vi "BB_Remote Sense Test_v3.vi"(7 "error in (no error)":errorcluster, 10 "ControlBoard VISA":refnum<visa-resource-name>="ControlBoard") -> (0 "error out":errorcluster, 2 "Voltage Readings":dbl[][](array[numeric]), 3 "Pass?":bool)   [LabVIEW 2022 SP3]
panel:
  in  "RemoteSenseRelayTask":refnum<k21>="BTS_RemoteSenseRelays"
  out "Message OUT":string
  out "MSE Array":dbl[](array[numeric])
  in  "Message IN":string
  out "Control Board OUT":refnum<visa-resource-name>
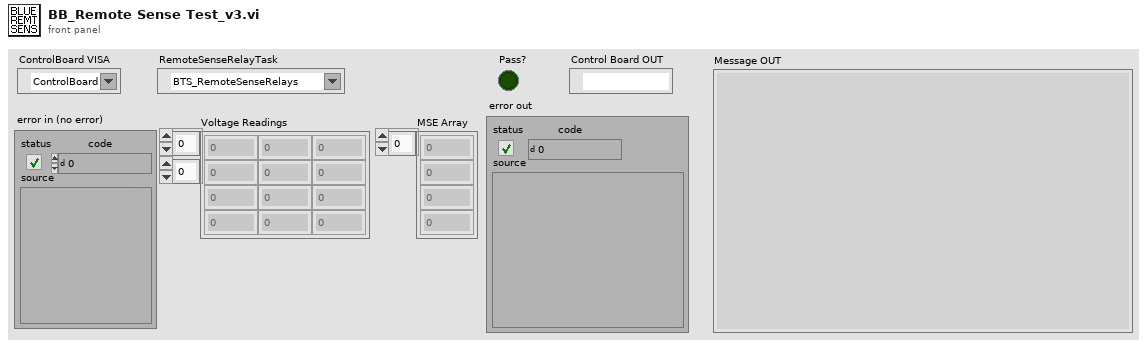
[diagram p1: front panel]
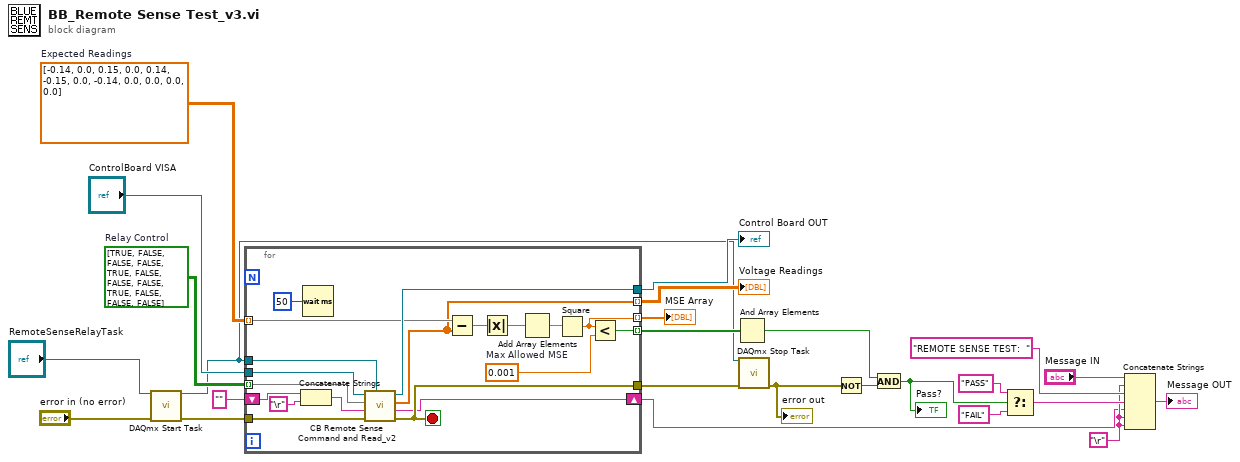
[diagram p0: block diagram]
diagram:
  w7 = dbl[][] [[-0.14, 0.0, 0.15], [0.0, 0.14, -0.15], [0.0, -0.14, 0.0], [0.0, 0.0, 0.0]]  # Expected Readings
  w13 = "\r"
  w23 = bool[][] [[TRUE, FALSE, FALSE], [FALSE, TRUE, FALSE], [FALSE, FALSE, TRUE], [FALSE, FALSE, FALSE]]  # Relay Control
  n1 = call "DAQmx Start Task.vi"("task/channels in"="RemoteSenseRelayTask", "error in"="error in (no error)") -> ("task out"=w1:refnum<k21>, "error out"=w4:errorcluster)  [unwired: 12 in]
  n2 = for {
    tunnel: [w42] -> w3
    tunnel: [w44] -> w25
    tunnel: w4 -> [w43]
    tunnel: w7 -> [w39] mode=indexing
    tunnel: [w36] -> w24 mode=indexing
    tunnel: w23 -> [w35] mode=indexing
    tunnel: [w34] -> w20 mode=indexing
    tunnel: [w33] -> w19 mode=indexing
    shift-right: [w32] -> w11
    shift-left: "" -> [w31]
    tunnel: "ControlBoard VISA" -> [w27]
    tunnel: w1 -> [w26]
    stop <- w42 stop-if-true
    w37 = 0.001  # Max Allowed MSE
    n3 = Concatenate Strings(w31, "\r") -> (w30:string)
    n4 = Wait (ms)(milliseconds to wait=u32 50) -> ()  [unwired: 1 out]
    n5 = call "CB Remote Sense Command and Read_v2.vi"("RemoteSenseRelayTask"=w26, "error in (no error)"=w43, "Message IN"=w30, "Relay Control"=w35, "ControlBoard VISA"=w27) -> ("error out"=w42:errorcluster, "Message OUT"=w32:string, "Voltage Array"=w34:dbl[], "Control Board OUT"=w44:refnum<visa-resource-name>)  [unwired: 3 in]
    n6 = Subtract(x=w39, y=w34) -> (x-y=w41:dbl[])
    n7 = Absolute Value(x=w41) -> (abs(x)=w40:dbl[])
    n8 = Add Array Elements(numeric array=w40) -> (sum=w38:dbl)
    n9 = Square(x=w38) -> (x^2=w33:dbl)
    n10 = Less?(x=w33, y=w37) -> (x < y?=w36:bool)
  }
  "Voltage Readings" <- w20
  "MSE Array" <- w19
  "Control Board OUT" <- w25
  n11 = And Array Elements(Boolean array=w24) -> (logical AND=w22:bool)
  n12 = call "DAQmx Stop Task.vi"("task/channels in"=w1, "error in"=w3) -> ("error out"=w2:errorcluster)  [unwired: 12 in, 1 out]
  "error out" <- w2
  n13 = Not(x=w2) -> (.not. x?=w21:bool)
  n14 = And(x=w22, y=w21) -> (x .and. y?=w12:bool)
  "Pass?" <- w12
  n15 = Select(t="PASS", s=w12, f="FAIL") -> (s? t:f=w17:string)
  n16 = Concatenate Strings("Message IN", w13, "REMOTE SENSE TEST:  ", w17, w11, w13, w13) -> (→"Message OUT":string)
